vi "GetLastModified.vi"(3 "error in":errorcluster, 4 "filenames":string[](array[string]), 5 "SearchDir":path) -> (0 "error out":errorcluster, 1 "last mod":timestamp, 2 "Path":path)   [LabVIEW 2015]
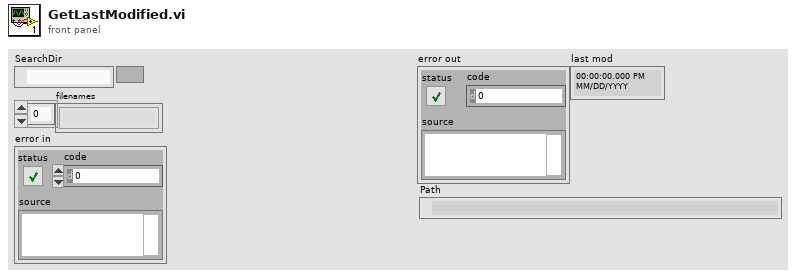
[diagram p1: front panel]
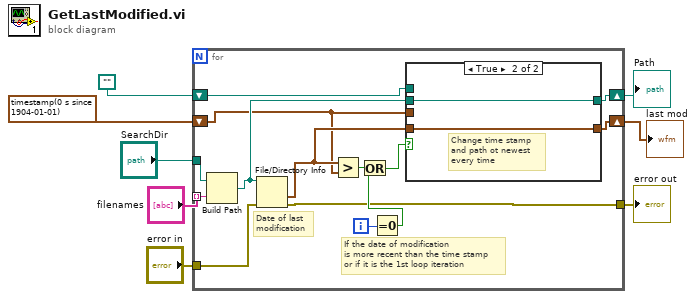
[diagram p0: block diagram]
diagram:
  n1 = for {
    tunnel: "filenames" -> [w14] mode=indexing
    tunnel: "SearchDir" -> [w22]
    shift-right: [w18] -> w2
    shift-left: timestamp(0 s since 1904-01-01) ("last mod 2") -> [w9]
    shift-right: [w17] -> w1
    shift-left: path "" -> [w15]
    tunnel: "error in" -> [w12]
    tunnel: [w11] -> w3
    i -> [w20]
    # "If the date of modification\nis more recent than the time stamp\nor if it is the 1st loop iteration"
    # "Date of last\nmodification"
    n2 = Build Path(base path=w22, name or relative path=w14) -> (appended path=w13:path)
    n3 = File/Directory Info(path=w13, error in=w12) -> (last mod=w10:timestamp, error out=w11:errorcluster)  [unwired: 5 out]
    n4 = Greater?(x=w10, y=w9) -> (0:w21:bool)
    n5 = Equal To 0?(x=w20) -> (x = 0?=w19:bool)
    n6 = Or(x=w21, y=w19) -> (x .or. y?=w16:bool)
    n7 = case shown="True" w16 {
      tunnel: w9 -> [w24 _]
      tunnel: w10 -> [_ w26]
      tunnel: w13 -> [_ w25]
      tunnel: [w23 w25] -> w17
      tunnel: w15 -> [w23 _]
      tunnel: [w24 w26] -> w18
      frame False {
        # "save the same time stamp \nand path as before"
      }
      frame True {
        # "Change time stamp\nand path ot newest \nevery time"
      }
    }
  }
  "error out" <- w3
  "last mod" <- w2
  "Path" <- w1
